vi "# giro de un motor.vi"() -> ()   [LabVIEW 2013]
uses:
  <vilib>/LabVIEW Interface for Arduino/Type Defs/Pin Mode.ctl
  <vilib>/LabVIEW Interface for Arduino/LabVIEW Interface for Arduino.lvlib
panel:
  out "Waveform Chart":dbl(graph)
  in  "Boolean 2":bool
  in  "Boolean":bool
  in  "stop":bool
  in  "Slide":dbl(slide) scale=0.0..255.0
  in  "PWM Pin (3)":u8=3
  in  "Pin Mode (Input) 2":T1
  in  "Digital I/O Pin":u8
  in  "Pin Mode (Input)":T1
  in  "Digital I/O Pin (0)":u8
  in  "VISA resource":refnum<visa-resource-name>
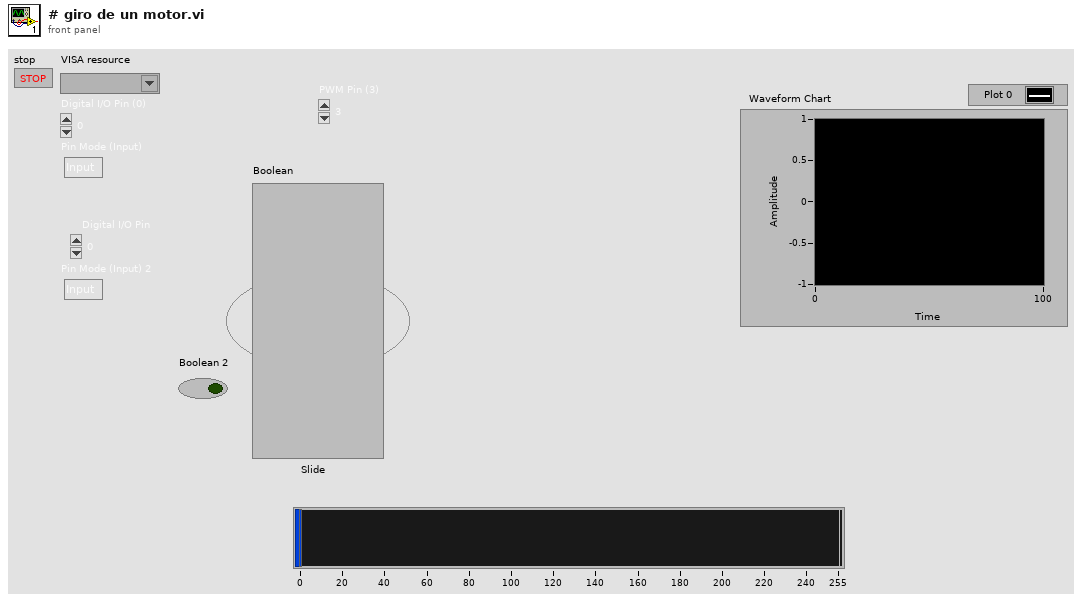
[diagram p1: front panel]
types:
  T1 = typedef "LabVIEW Interface for Arduino.lvlib/Pin Mode.ctl" = enum8{"Input", "Output"}
  T2 = typedef "LabVIEW Interface for Arduino.lvlib/Arduino Resource.ctl" = cluster{"VISA resource":refnum<visa-resource-name>, "Board Type":T3, "Connection Type":enum8{"USB / Serial"}, "Bytes Per Packet (15)":u8}
  T3 = typedef "LabVIEW Interface for Arduino.lvlib/Board Type.ctl" = enum16{"Uno", "Dimuelanove w/Atmega 328", "Mega 2560"}
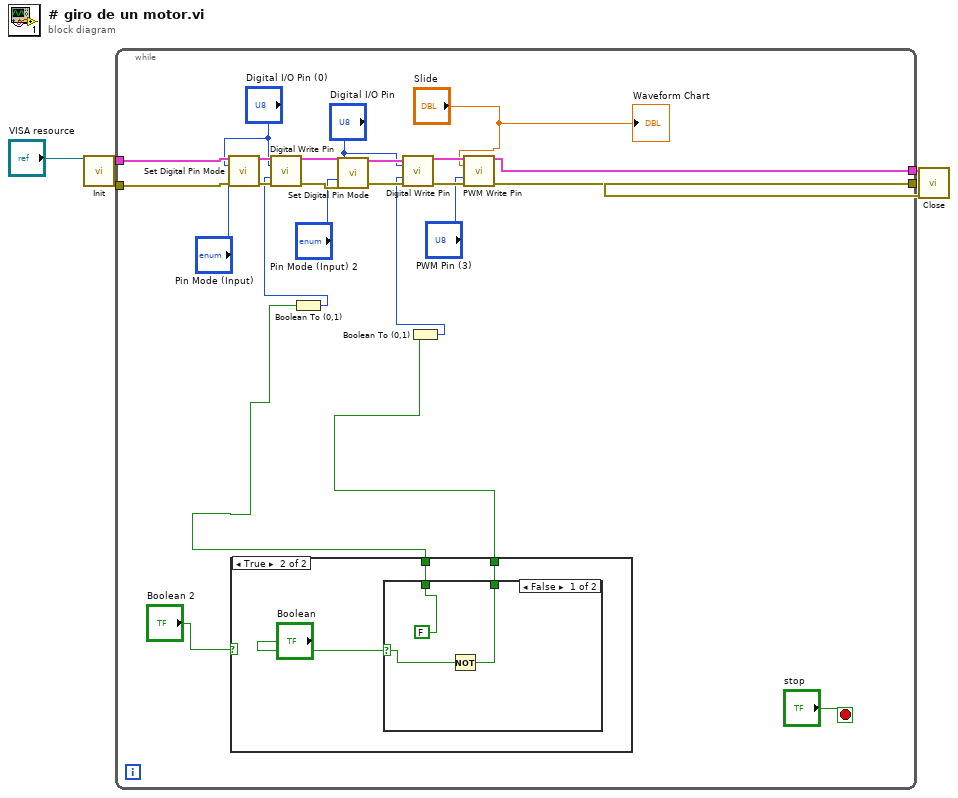
[diagram p0: block diagram]
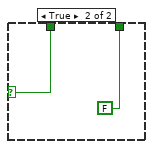
[diagram p3: hidden frame]
diagram:
  n1 = call <vilib>:"Init.vi"("VISA resource"="VISA resource") -> ("Arduino Resource"=w5:T2, "error out"=w2:errorcluster)  [unwired: 17 in]
  n2 = while {
    tunnel: w5 -> [w29]
    tunnel: [w24] -> w4
    tunnel: [w23] -> w3
    tunnel: w2 -> [w18]
    stop <- "stop" stop-if-true
    n3 = call <vilib>:"Set Digital Pin Mode.vi"("Arduino Resource"=w29, "Digital I/O Pin"="Digital I/O Pin (0)", "Pin Mode (Input)"="Pin Mode (Input)", "error in"=w18) -> ("Arduino Resource"=w28:T2, "error out"=w19:errorcluster)  [unwired: 10 in]
    n4 = case shown="True" "Boolean 2" {
      selector: "Boolean 2" -> [w30 _]
      tunnel: [w30 w33] -> w9
      tunnel: [w30 w32] -> w8
      frame False {
      }
      frame True {
        n5 = case shown="False" "Boolean" {
          selector: "Boolean" -> [w35 w38]
          tunnel: [FALSE w38] -> w33
          tunnel: [w34 FALSE] -> w32
          frame False {
            n6 = Not(x=w35) -> (.not. x?=w34:bool)
          }
          frame True {
          }
        }
      }
    }
    n7 = Boolean To (0,1)(Boolean=w9) -> (0, 1=w15:i16)
    n8 = call <vilib>:"Digital Write Pin.vi"("Arduino Resource"=w28, "Digital I/O Pin (0)"="Digital I/O Pin (0)", "Value (0)"=w15, "error in"=w19) -> ("Arduino Resource"=w27:T2, "error out"=w20:errorcluster)  [unwired: 10 in]
    n9 = call <vilib>:"Set Digital Pin Mode.vi"("Arduino Resource"=w27, "Digital I/O Pin"="Digital I/O Pin", "Pin Mode (Input)"="Pin Mode (Input) 2", "error in"=w20) -> ("Arduino Resource"=w26:T2, "error out"=w21:errorcluster)  [unwired: 10 in]
    n10 = Boolean To (0,1)(Boolean=w8) -> (0, 1=w14:i16)
    n11 = call <vilib>:"Digital Write Pin.vi"("Arduino Resource"=w26, "Digital I/O Pin (0)"="Digital I/O Pin", "Value (0)"=w14, "error in"=w21) -> ("Arduino Resource"=w25:T2, "error out"=w22:errorcluster)  [unwired: 10 in]
    n12 = call <vilib>:"PWM Write Pin.vi"("Arduino Resource"=w25, "Duty Cycle (0 - 255)"="Slide", "PWM Pin (3)"="PWM Pin (3)", "error in"=w22) -> ("Arduino Resource"=w24:T2, "error out"=w23:errorcluster)  [unwired: 10 in]
    "Waveform Chart" <- "Slide"
  }
  n13 = call <vilib>:"Close.vi"("Arduino Resource"=w4, "error in"=w3) -> ()  [unwired: 13 in, 1 out]
